vi "fetching _data.vi"(8 "table":string, 9 "value_in_the_field_to_find":string, 10 "select_the_field_to_search":string(combo), 11 "database_link":path) -> (2 "data":cluster{string, i32, dbl}[](array[cluster]), 3 "error out":errorcluster)   [LabVIEW 2019]
uses:
  <vilib>/addons/database/Connection.llb/DB Tools Open Connec (Path).vi
  <vilib>/addons/database/_DB Variant To Data/Database Variant To Data.xnode
  <vilib>/addons/database/NI_Database_API.lvlib
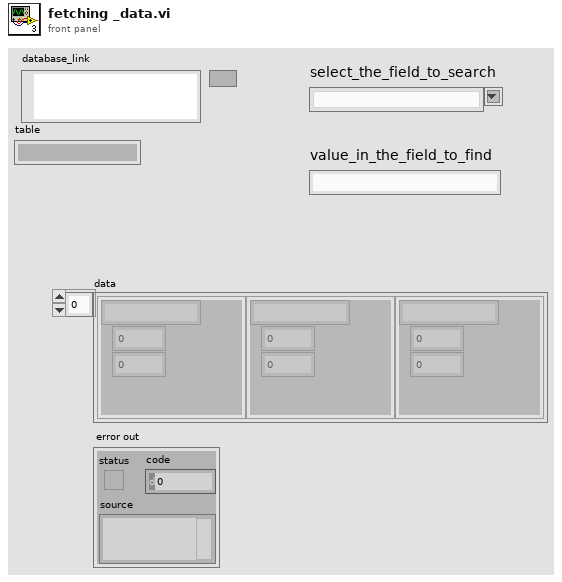
[diagram p1: front panel]
types:
  T1 = typedef "NI_Database_API.lvlib/Conn ObjectReference.ctl" = refnum<k1>
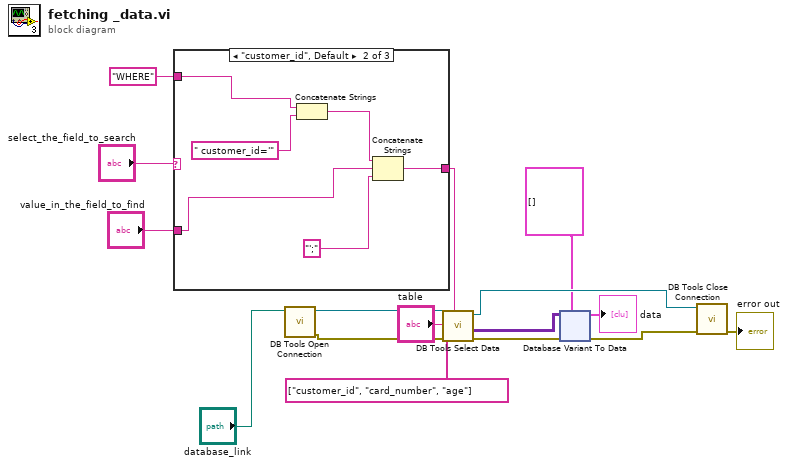
[diagram p0: block diagram]
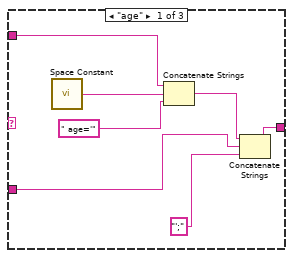
[diagram p2: hidden frame]
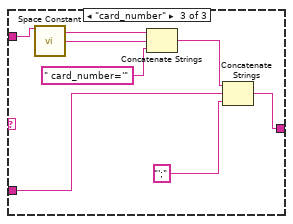
[diagram p3: hidden frame]
diagram:
  n1 = case shown="\"customer_id\", Default" "select_the_field_to_search" {
    tunnel: "WHERE" -> [w20 w29 w33]
    tunnel: [w18 w26 w31] -> w4
    tunnel: "value_in_the_field_to_find" -> [w17 w25 w30]
    frame "age" {
      n2 = call <vilib>:"Space Constant.vi"() -> ("String"=w23:string)
      n3 = Concatenate Strings(w20, w23, " age='") -> (w21:string)
      n4 = Concatenate Strings(w21, w17, "';") -> (w18:string)
    }
    frame "customer_id", Default {
      n5 = Concatenate Strings(w29, " customer_id='") -> (w28:string)
      n6 = Concatenate Strings(w28, w25, "';") -> (w26:string)
    }
    frame "card_number" {
      n7 = call <vilib>:"Space Constant.vi"() -> ("String"=w36:string)
      n8 = Concatenate Strings(w33, w36, " card_number='") -> (w34:string)
      n9 = Concatenate Strings(w34, w30, "';") -> (w31:string)
    }
  }
  n10 = call-poly <vilib>:"DB Tools Open Connection.vi"("connection information"="database_link") -> ("error out"=w14:errorcluster, "connection reference"=w15:T1)  [unwired: 7 in]
  n11 = call <vilib>:"DB Tools Select Data.vi"("condition"=w4, "error in (no error)"=w14, "columns"=string[] ["customer_id", "card_number", "age"], "table"="table", "connection reference"=w15) -> ("error out"=w12:errorcluster, "data"=w13:variant[][], "connection reference out"=w10:T1)  [unwired: 1 in]
  n12 = xnode "Database Variant To Data"("database variant"=w13, "error in (no error)"=w12, "type"=cluster{string, i32, dbl}[] []) -> ("data"=→"data":cluster{string, i32, dbl}[], "error out"=w11:errorcluster)
  n13 = call <vilib>:"DB Tools Close Connection.vi"("error in (no error)"=w11, "connection reference"=w10) -> ("error out"=→"error out":errorcluster)  [unwired: 5 in]
